vi "(SubVI)Update Log_Delay with Log.vi"(5 "Log Ref":refnum<vi>, 10 "error in (no error)":errorcluster caption="에러 입력(에러 없음)", 11 "Delay (ms)":u32) -> (2 "error out":errorcluster caption="에러 출력", 3 "Log":string)   [LabVIEW 2020]
uses:
  3ca1c173-4ea7-47a3-b0d4-f075d2f9824e.vi
panel:
  # "(SubVI)Delay with Log.vi By hspark\n\nDescription : 에러라인 연결로 데이터 흐름 사이에 간편하게 사용할 수 있는 Delay. Log Ref 입력 시 Log가 자동으로 추가됨.\n\nInput : \n1. Delay (ms) : Delay 시간. 0 입력 시 무시됨.\n2. Log Ref : Log를 남길 문자열 인디케이터 참조. 입력하지 않은 경우 Log를 남기지 않음. (Log 출력은 유지)\n\nOutput : \n1. Log : 생성된 Log 문자열\n\nLabVIEW Version : 2020 SP1 이상\n\nNote :\n\nUpdate : 2021.10.06"
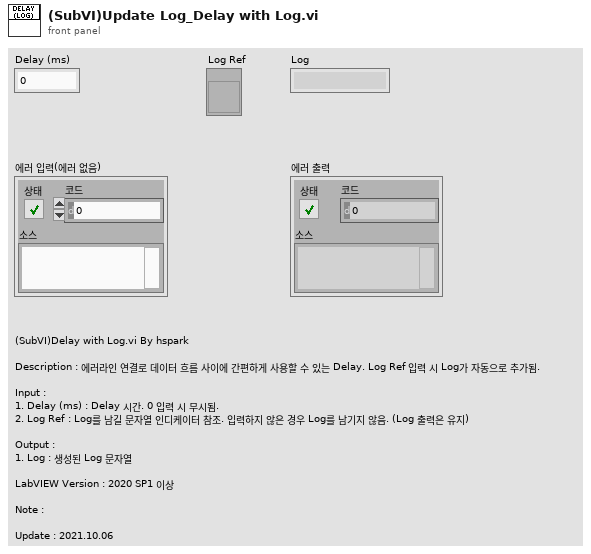
[diagram p1: front panel]
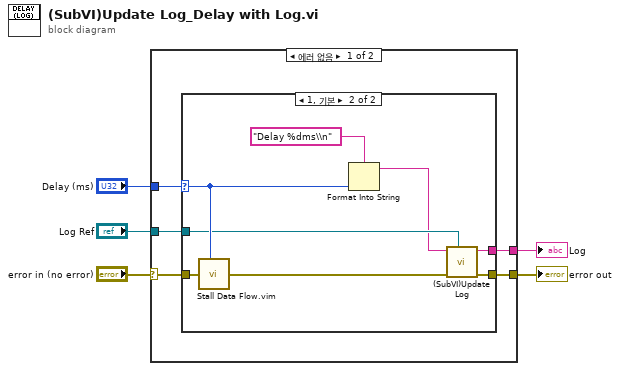
[diagram p0: block diagram]
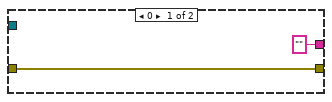
[diagram p2: hidden frame]
diagram:
  n1 = case shown="에러 없음" "error in (no error)" {
    selector: "error in (no error)" -> [w9 w21]
    tunnel: "Delay (ms)" -> [w10 _]
    tunnel: [w6 _] -> w4
    tunnel: [w8 w21] -> w2
    tunnel: "Log Ref" -> [w7 _]
    frame No Error {
      n2 = case shown="1, 기본" w10 {
        selector: w10 -> [_ w20]
        tunnel: w9 -> [w11 w19]
        tunnel: [w11 w17] -> w8
        tunnel: w7 -> [_ w16]
        tunnel: ["" ("Log out") w14] -> w6
        frame 0 {
        }
        frame 1, Default {
          n3 = call "Stall Data Flow.vim"("value in"=w19, "milliseconds to wait"=w20) -> ("value out"=w18:errorcluster)  [unwired: 1 out]
          n4 = Format Into String(format string="Delay %dms\\n" ("포맷 문자열"), w20) -> (resulting string=w15:string)  [unwired: 2 in, 1 out]
          n5 = call "(SubVI)Update Log.vi"("Log Ref"=w16, "error in (no error)"=w18, "Log"=w15) -> ("error out"=w17:errorcluster, "Log out"=w14:string)  [unwired: 7 in]
        }
      }
    }
    frame Error {
    }
  }
  "Log" <- w4
  "error out" <- w2
